vi "Demo.vi"() -> ()   [LabVIEW 2020, in "Tag Tree.lvclass"]
uses:
  Tag Tree.lvclass
panel:
  out "Selected Tags":string[](array[string])
  in  "Tree":string[](tree)
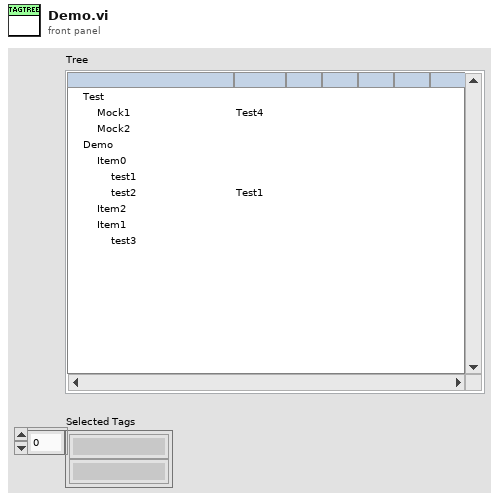
[diagram p1: front panel]
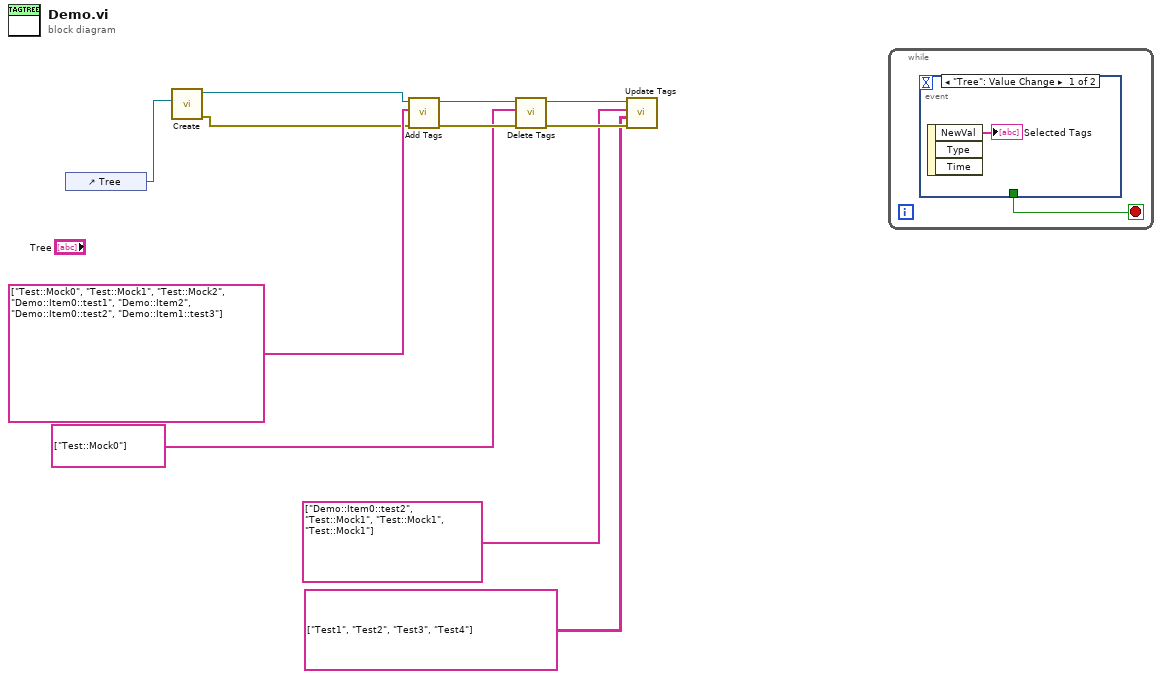
[diagram p0: block diagram]
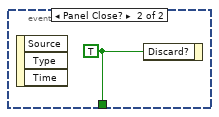
[diagram p2: hidden frame]
diagram:
  n1 = control-ref of="Tree"() -> (w1:refnum<vi>)
  n2 = call "Create.vi"("TreeControl in"=w1) -> ("error out"=w9:errorcluster, "Tag Tree out"=w11:refnum<class "Tag Tree.lvclass">)  [unwired: 9 in]
  n3 = call "Add Tags.vi"("error in (no error)"=w9, "Tag"=string[] ["Test::Mock0", "Test::Mock1", "Test::Mock2", "Demo::Item0::test1", "Demo::Item2", "Demo::Item0::test2", "Demo::Item1::test3"], "Tag Tree In"=w11) -> ("error out"=w7:errorcluster, "Tag Tree Out"=w8:refnum<class "Tag Tree.lvclass">)  [unwired: 7 in]
  n4 = call "Delete Tags.vi"("error in (no error)"=w7, "Tag"=string[] ["Test::Mock0"], "Tag Tree In"=w8) -> ("error out"=w5:errorcluster, "Tag Tree Out"=w4:refnum<class "Tag Tree.lvclass">)  [unwired: 7 in]
  n5 = call "Update Tags.vi"("error in (no error)"=w5, "Child Text"=string[][] [["Test1"], ["Test2"], ["Test3"], ["Test4"]], "Tag"=string[] ["Demo::Item0::test2", "Test::Mock1", "Test::Mock1", "Test::Mock1"], "Tag Tree In"=w4) -> ()  [unwired: 6 in, 2 out]
  n6 = while {
    stop <- w12 stop-if-true
    n7 = event shown="[0] \"Tree\": Value Change" {
      selector: _ -> [_ _]
      dyn-events: _ -> [_ _]
      timeout: _ -> [_ _]
      tunnel: [_ w14] -> w12
      event "Tree": Value Change {
        n8 = event-data() -> ("NewVal"=→"Selected Tags":string[])  [unwired: 1 in, 2 out]
      }
      event Panel Close? {
        w14 = TRUE ("Discard?")
        n9 = event-data() -> ()  [unwired: 1 in, 3 out]
        n10 = event-data ("Event Filter Node")("Discard?"=w14) -> ()  [unwired: 1 in, 1 out]
      }
    }
  }
